vi "test-globallog for CSM error.vi"(8 "error in (no error)":errorcluster, 11 "TestCase in":refnum<class "testcase-globalLog.lvclass">) -> (0 "error out":errorcluster, 3 "TestCase out":refnum<class "testcase-globalLog.lvclass">)   [LabVIEW 2017, in "testcase-globalLog.lvclass"]
uses:
  testcase-globalLog.lvclass
  src/user.lib/_NEVSTOP/Communicable State Machine(CSM)/_Support/Typedef/_CSM_GlobalLog_MSG.ctl
  src/user.lib/_NEVSTOP/Communicable State Machine(CSM)/_Support/Typedef/_CSM_Response Source Message.ctl
  src/user.lib/_NEVSTOP/Communicable State Machine(CSM)/_Support/Typedef/_CSM_GlobalLog_MSG_TYPE.ctl
  61f80922-628e-48dd-9b7e-09b6add618c8.vi
  <vilib>/addons/_JKI Toolkits/VI Tester/TestCase.llb/TestCase.lvclass
  src/user.lib/_NEVSTOP/Communicable State Machine(CSM)/Communicable State Machine.lvlib
  C:/Program Files (x86)/National Instruments/LabVIEW 2017/vi.lib/addons/_JKI Toolkits/VI Tester/TestCase.llb/TestCase.lvclass
panel:
  out "State History":string
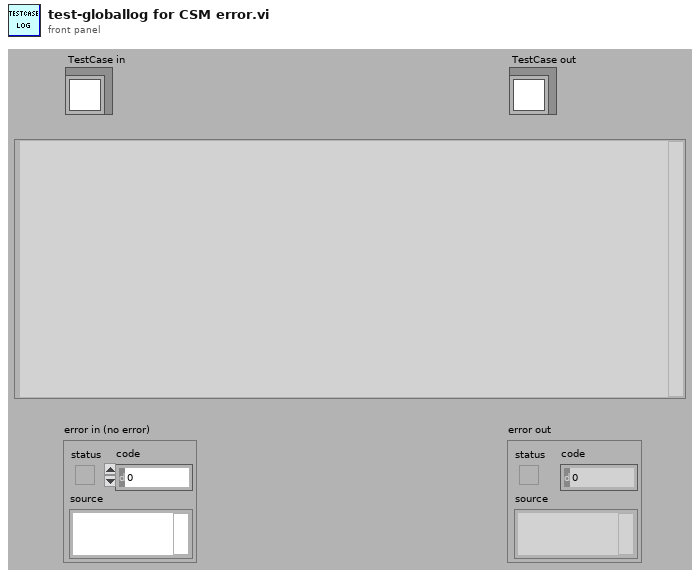
[diagram p1: front panel]
types:
  T1 = cluster{"threashold(#/s)":dbl, "Check Peroid(s)":dbl}
  T2 = typedef "Communicable State Machine.lvlib/_CSM_GlobalLog_MSG.ctl" = cluster{"Name (\"\" to Use UUID)":string, "Current State":string, "Arguments":string, "Source Message":T3, "Source Module":string, "Complete(T)/Start(F)":bool, "LogType":T4, "Time Stamp":timestamp}
  T3 = typedef "Communicable State Machine.lvlib/_CSM_Response Source Message.ctl" = cluster{"‘State":string, "’Arguments":string, "’Error":errorcluster}
  T4 = typedef "Communicable State Machine.lvlib/_CSM_GlobalLog_MSG_TYPE.ctl" = enum16{"User Log", "State Change", "Status", "Interrupt", "Register", "Unregister", "Error Log", "Module Created", "Module Destroyed", "Async Message", "No-Rep Async Message", "Sync Message", "AsyncMsg Complete", "SyncMsg Complete"}
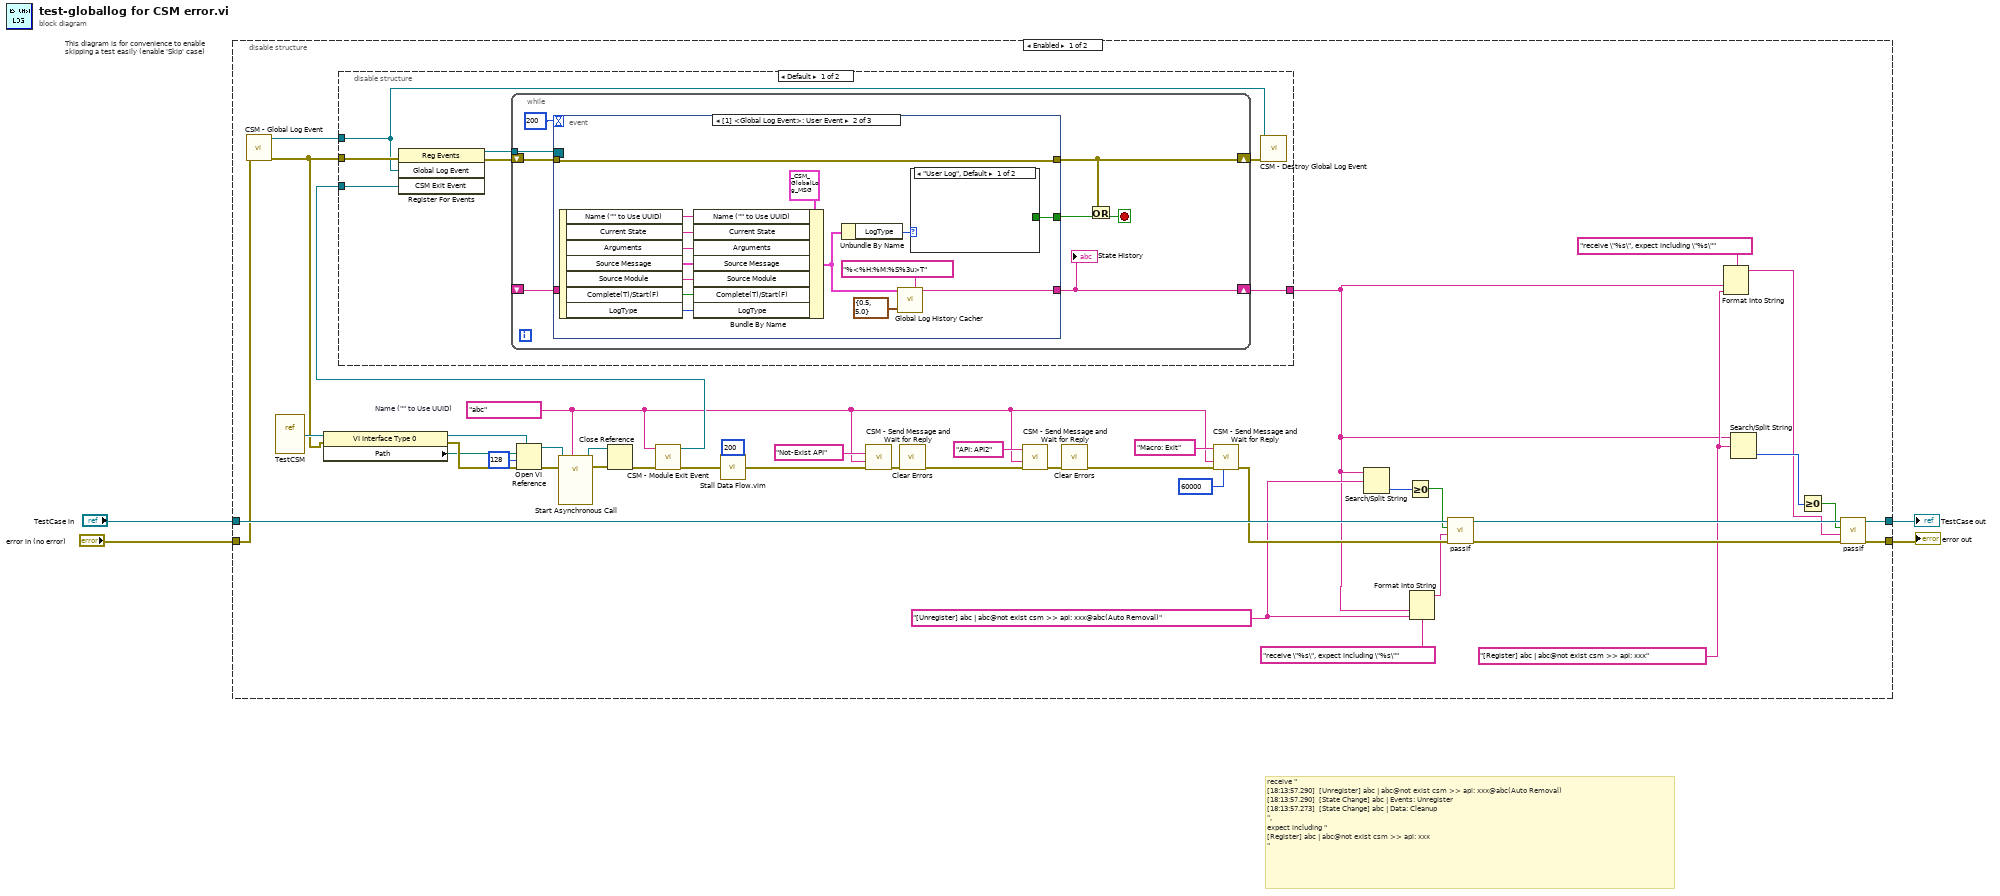
[diagram p0: block diagram]
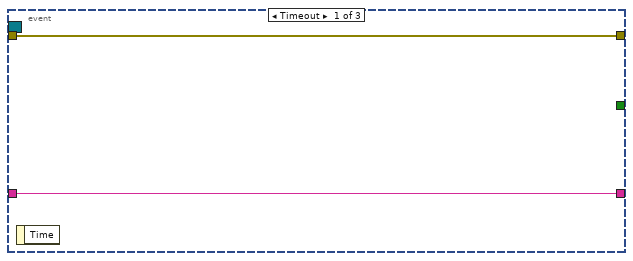
[diagram p2: hidden frame]
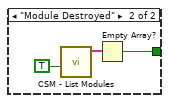
[diagram p3: hidden frame]
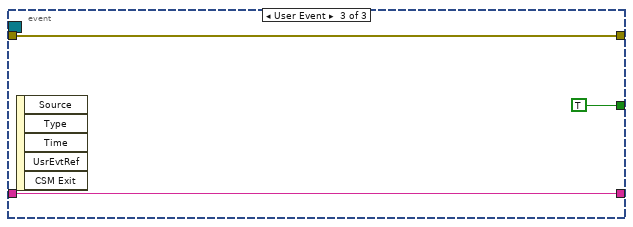
[diagram p4: hidden frame]
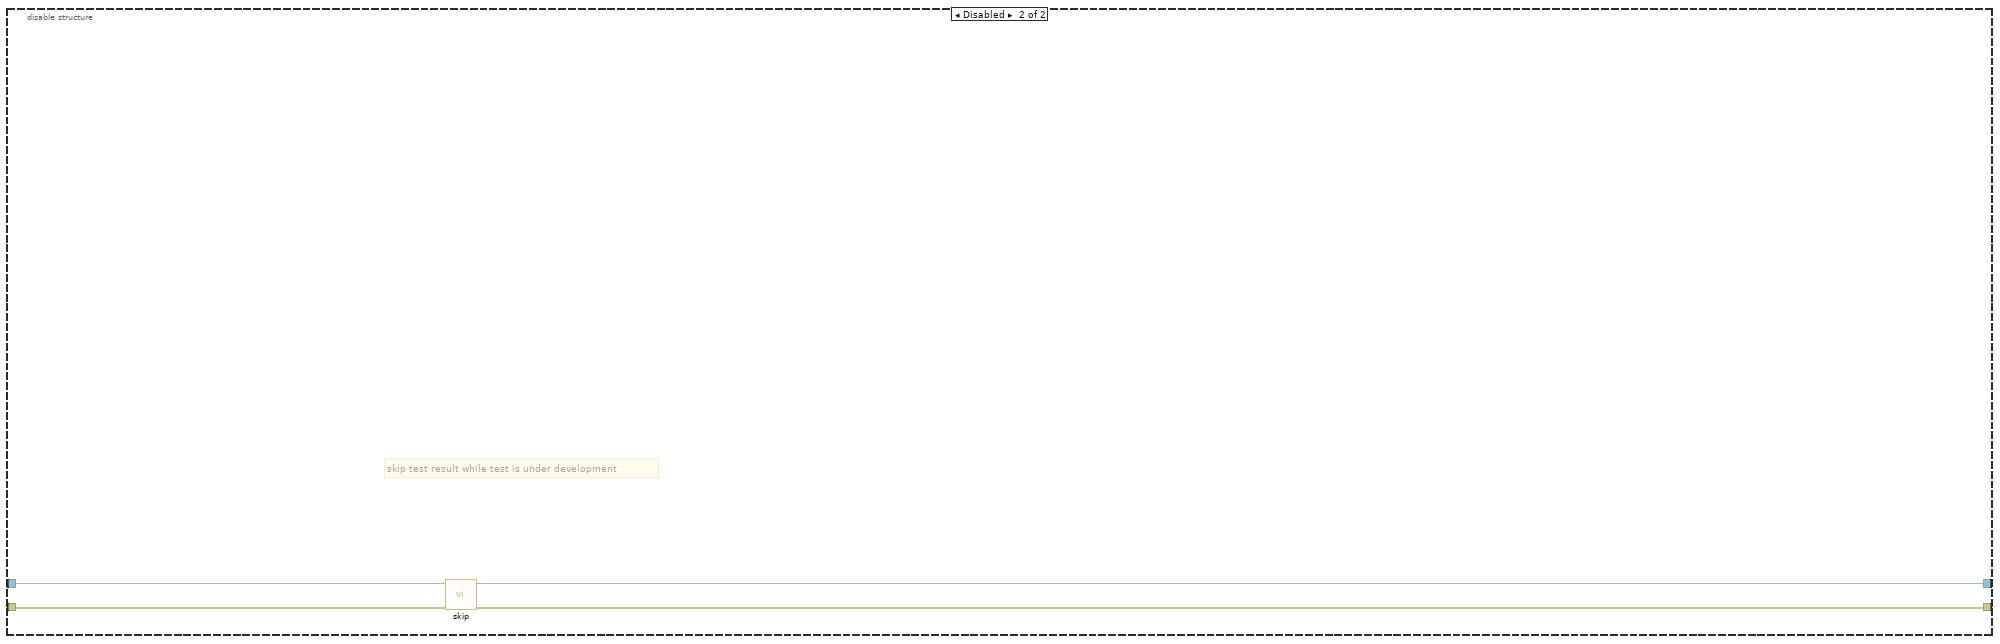
[diagram p6: hidden frame]
diagram:
  # "receive \"\n[18:13:57.290]  [Unregister] abc | abc@not exist csm >> api: xxx@abc(Auto Removal)\n[18:13:57.290]  [State Change] abc | Events: Unregister\n[18:13:57.273]  [State Change] abc | Data: Cleanup\n\", \nexpect including \"\n[Register] abc | abc@not exist csm >> api: xxx\n\""
  n1 = disable-structure "This diagram is for convenience to enable skipping a test easily (enable 'Skip' case)" shown="Enabled" {
    disable-tunnel: "TestCase in" -> [w47 w89]
    disable-tunnel: [w21 w87] -> w1
    disable-tunnel: [w20 w88] -> w3
    disable-tunnel: "error in (no error)" -> [w6 w86]
    frame Enabled {
      w11 = "[Register] abc | abc@not exist csm >> api: xxx" ("string")
      w14 = "[Unregister] abc | abc@not exist csm >> api: xxx@abc(Auto Removal)" ("string")
      w25 = "abc"  # Name ("" to Use UUID)
      n2 = call "CSM - Global Log Event.vi"("Error In"=w6) -> ("error out"=w7:errorcluster, "Global Log Event"=w8:refnum<user-event>)  [unwired: 9 in]
      n3 = vi-ref "TestCSM.vi"() -> (w39:refnum<vi>)
      n4 = property class="VI Interface Type 0"(reference=w39, error in=w7) -> (reference out=w43:refnum<vi>, error out=w41:errorcluster, "Path"=w40:path)
      n5 = Open VI Reference(type specifier VI Refnum (for type only)=w43, vi path=w40, options=128, error in (no error)=w41) -> (vi reference=w42:refnum<vi>, error out=w38:errorcluster)  [unwired: 2 in]
      n6 = call-by-ref "Start Asynchronous Call"(reference=w42, error in=w38, "Name(\"\" to use uuid)"=w25) -> (reference out=w45:refnum<vi>, error out=w44:errorcluster)  [unwired: 11 in]
      n7 = Close Reference(reference=w45, error in (no error)=w44) -> (error out=w37:errorcluster)
      n8 = call "CSM - Module Exit Event.vi"("Error In"=w37, "Name (\"\" to Use UUID) In"=w25) -> ("error out"=w36:errorcluster, "CSM Exit Event"=w35:refnum<user-event>)  [unwired: 7 in, 1 out]
      n9 = disable-structure shown="Default" {
        disable-tunnel: w35 -> [w51 _]
        disable-tunnel: [w50 _] -> w9
        disable-tunnel: w7 -> [w49 _]
        disable-tunnel: w8 -> [w48 _]
        frame condition #0 (active) {
          n10 = register-events(error in=w49, w48, w51) -> (reference out=w53:refnum<event-registration>, error out=w54:errorcluster)  [unwired: 1 in]
          n11 = while {
            tunnel: w53 -> [w62]
            shift-right: [w59] -> w52
            shift-left: w54 -> [w61]
            shift-right: [w56] -> w50
            shift-left: _ -> [w55]
            stop <- w60 stop-if-true
            n12 = event shown="[1] <Global Log Event>: User Event" {
              selector: w62 -> [_ _ _]
              dyn-events: _ -> [_ _ _]
              timeout: 200 -> [_ _ _]
              tunnel: w61 -> [w64 w79 w85]
              tunnel: [w64 w79 w85] -> w59
              tunnel: [_ w68 TRUE ("empty?")] -> w58
              tunnel: [w63 w65 w83] -> w56
              tunnel: w55 -> [w63 _ w83]
              event Timeout {
                n13 = event-data() -> ()  [unwired: 1 in, 1 out]
              }
              event User Event {
                n14 = event-data() -> ("Name (\"\" to Use UUID)"=w78:string, "Current State"=w77:string, "Arguments"=w76:string, "Source Message"=w75:T3, "Source Module"=w74:string, "Complete(T)/Start(F)"=w73:bool, "LogType"=w72:T4)  [unwired: 1 in]
                n15 = Bundle By Name(cluster=T2 {"Name (\"\" to Use UUID)"="", "Current State"="", "Arguments"="", "Source Message"={"‘State"="", "’Arguments"="", "’Error"={"status"=FALSE, "code"=0, "source"=""}}, "Source Module"="", "Complete(T)/Start(F)"=FALSE, "LogType"=enum."State Change", "Time Stamp"=timestamp(0 s since 1904-01-01)} ("Cross CSM Data"), "Name (\"\" to Use UUID)"=w78, "Current State"=w77, "Arguments"=w76, "Source Message"=w75, "Source Module"=w74, "Complete(T)/Start(F)"=w73, "LogType"=w72) -> (w70:T2)
                n16 = Unbundle By Name(w70) -> ("LogType"=w69:T4)
                n17 = call "Global Log History Cacher.vi"("Global Log Data"=w70, "Time Format String"="%<%H:%M:%S%3u>T" ("Time format string"), "Settings"=T1 {"threashold(#/s)"=0.5, "Check Peroid(s)"=5.0}) -> ("String Cache"=w65:string)  [unwired: 12 in]
                n18 = case shown="\"User Log\", Default" w69 {
                  tunnel: [_ w80] -> w68
                  frame "User Log", Default {
                  }
                  frame "Module Destroyed" {
                    n19 = call "CSM - List Modules.vi"("With Nodes? (F)"=TRUE ("All?")) -> ("Module Names"=w82:string[])  [unwired: 9 in, 1 out]
                    n20 = Empty Array?(array=w82) -> (empty?=w80:bool)
                  }
                }
              }
              event User Event {
                n21 = event-data() -> ()  [unwired: 1 in, 5 out]
              }
            }
            "State History" <- w56
            n22 = Or(x=w59, y=w58) -> (x .or. y?=w60:bool)
          }
          n23 = call "CSM - Destroy Global Log Event.vi"("Error In"=w52, "CSM Global Log Event"=w48) -> ()  [unwired: 9 in, 1 out]
        }
        frame condition #1 {
        }
      }
      n24 = call "Stall Data Flow.vim"("value in"=w36, "milliseconds to wait"=u32 200) -> ("value out"=w31:errorcluster)  [unwired: 1 out]
      n25 = call "CSM - Send Message and Wait for Reply.vi"("Error In (No Error)"=w31, "Target Module"=w25, "State"="Not-Exist API") -> ("error out"=w30:errorcluster)  [unwired: 6 in, 2 out]
      n26 = call <vilib>:"Clear Errors.vi"("error in (no error)"=w30) -> ("error out"=w26:errorcluster)  [unwired: 5 in, 1 out]
      n27 = call "CSM - Send Message and Wait for Reply.vi"("Error In (No Error)"=w26, "Target Module"=w25, "State"="API: API2") -> ("error out"=w27:errorcluster)  [unwired: 6 in, 2 out]
      n28 = call <vilib>:"Clear Errors.vi"("error in (no error)"=w27) -> ("error out"=w24:errorcluster)  [unwired: 5 in, 1 out]
      n29 = call "CSM - Send Message and Wait for Reply.vi"("Response Timeout (-2 Using Global Settings)"=60000, "Error In (No Error)"=w24, "Target Module"=w25, "State"="Macro: Exit") -> ("error out"=w34:errorcluster)  [unwired: 5 in, 2 out]
      n30 = Search/Split String(string=w9, search string/char (-)=w14) -> (offset of match=w19:i32)  [unwired: 1 in, 2 out]
      n31 = Greater Or Equal To 0?(x=w19) -> (x >= 0?=w18:bool)
      n32 = Format Into String(format string="receive \"%s\", expect including \"%s\"", w9, w14) -> (resulting string=w13:string)  [unwired: 2 in, 1 out]
      n33 = call-dynamic "passIf.vi"("error in (no error)"=w34, "message (\"\")"=w13, "pass"=w18, "TestCase in"=w47) -> ("error out"=w23:errorcluster, "TestCase out"=w22:refnum<class "testcase-globalLog.lvclass">)  [unwired: 6 in]
      n34 = Format Into String(format string="receive \"%s\", expect including \"%s\"", w9, w11) -> (resulting string=w10:string)  [unwired: 2 in, 1 out]
      n35 = Search/Split String(string=w9, search string/char (-)=w11) -> (offset of match=w17:i32)  [unwired: 1 in, 2 out]
      n36 = Greater Or Equal To 0?(x=w17) -> (x >= 0?=w16:bool)
      n37 = call-dynamic "passIf.vi"("error in (no error)"=w23, "message (\"\")"=w10, "pass"=w16, "TestCase in"=w22) -> ("error out"=w20:errorcluster, "TestCase out"=w21:refnum<class "testcase-globalLog.lvclass">)  [unwired: 6 in]
    }
    frame Disabled {
      # "skip test result while test is under development"
      n38 = call <vilib>:"skip.vi"("error in (no error)"=w86, "TestCase in"=w89) -> ("error out"=w88:errorcluster, "TestCase out"=w87:refnum<class "testcase-globalLog.lvclass">)  [unwired: 8 in]
    }
  }
  "error out" <- w3
  "TestCase out" <- w1
